vi "Read Scan depth (mm).vi"(8 "error in (no error)":errorcluster, 11 "Spectrometer in":refnum<class "Spectrometer.lvclass">) -> (0 "error out":errorcluster, 2 "Scan depth (mm)":dbl=2.0, 3 "Spectrometer out":refnum<class "Spectrometer.lvclass">)   [LabVIEW 2017, in "Spectrometer.lvclass"]
uses:
  Spectrometer.lvclass
  Spectrometer.lvclass/Spectrometer.ctl
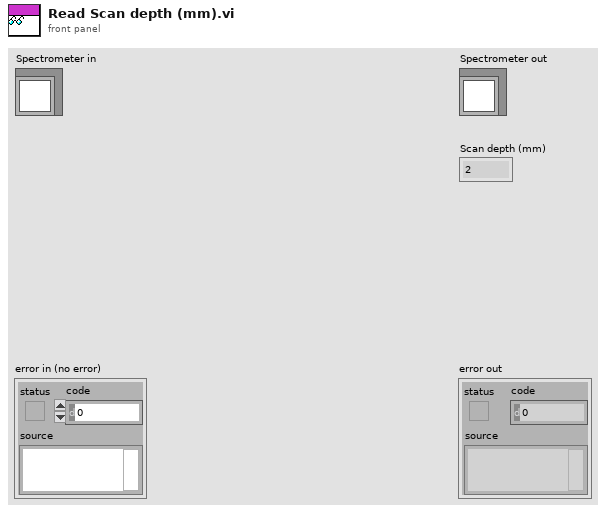
[diagram p1: front panel]
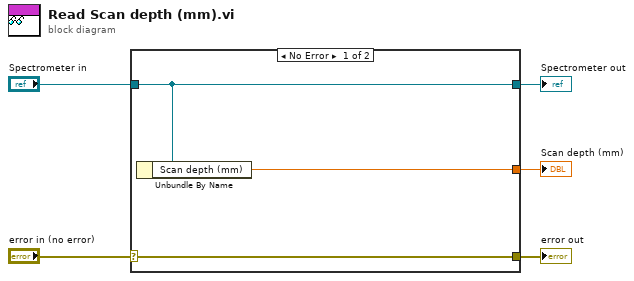
[diagram p0: block diagram]
diagram:
  n1 = case shown="No Error" "error in (no error)" {
    selector: "error in (no error)" -> [w8 w9]
    tunnel: [w8 w9] -> w4
    tunnel: [w7 w10] -> w2
    tunnel: "Spectrometer in" -> [w7 w10]
    tunnel: [w6 _] -> w1
    frame No Error {
      n2 = Unbundle By Name(w7) -> ("Scan depth (mm)"=w6:dbl)
    }
    frame Error {
    }
  }
  "error out" <- w4
  "Spectrometer out" <- w2
  "Scan depth (mm)" <- w1
